vi "GE 5565PIORC.Bit Manipulation.Create Mask (U64).vi"(10 "bit count (1)":i32=1, 11 "bit index (0)":i32) -> (3 "mask":u64 format="%016x")   [LabVIEW 2016, in "GE 5565PIORC.lvclass"]
doc: "This VI creates a mask that can be used to extract bits from a scalar starting at <B>bit index</B> and of length <B>bit count</B>."
uses:
  GE 5565PIORC.lvclass
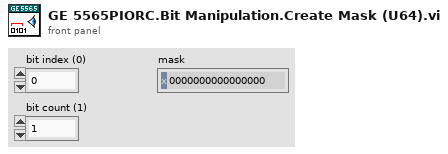
[diagram p1: front panel]
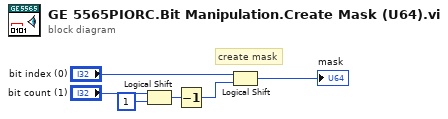
[diagram p0: block diagram]
diagram:
  # "create mask"
  n1 = Logical Shift(y="bit count (1)", x=u64 1) -> (x << y=w4:u64)
  n2 = Decrement(x=w4) -> (x-1=w3:u64)
  n3 = Logical Shift(y="bit index (0)", x=w3) -> (x << y=→"mask":u64)
